vi "DrawBuoy.vi"(2 "Array":dbl[][](array[numeric]), 3 "2D Picture":picture) -> (0 "new picture":picture)   [LabVIEW 2012]
doc: "Draws a magenta circle at the curretn (x,y) coordinates of the Robot in the current mission definition file.\nInputs:\nPicture to draw on\nCluster X\n y coordinates of robot\nOutput:\nmodified picture"
panel:
  # "Draws a circle at the current x,y coordinates of the robot"
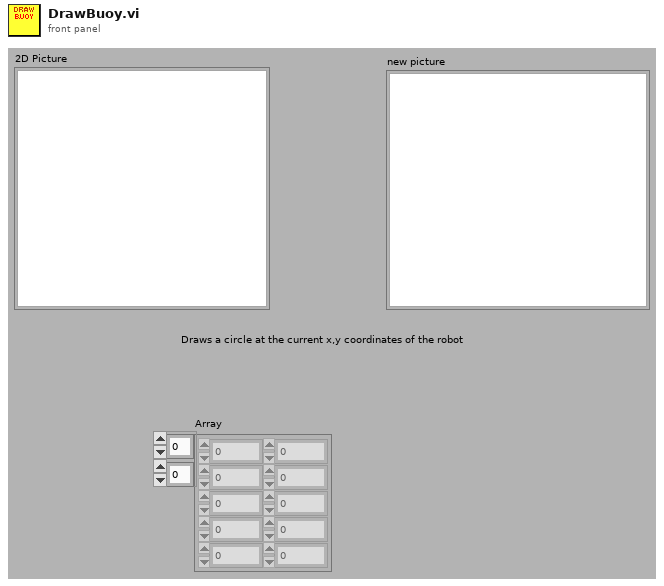
[diagram p1: front panel]
types:
  T1 = cluster{"Width":u16, "Style":enum32{"Solid", "Dash", "Dot", "DashDot", "DashDotDot"}}
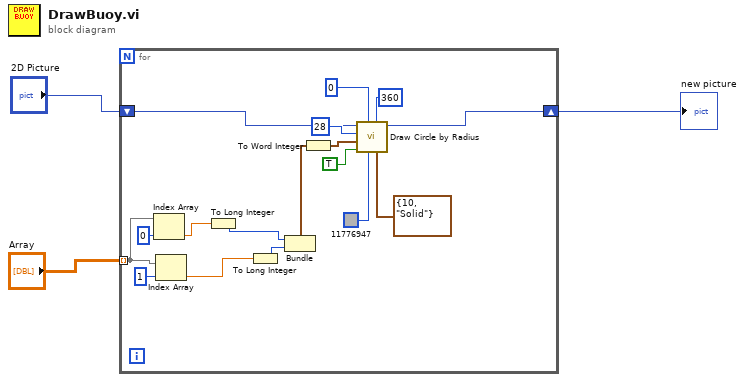
[diagram p0: block diagram]
diagram:
  n1 = for {
    shift-right: [w9] -> w2
    shift-left: "2D Picture" -> [w14]
    tunnel: "Array" -> [w6] mode=indexing
    n2 = Index Array(array=w6, index=0) -> (element=w5:dbl)
    n3 = Index Array(array=w6, index=1) -> (element=w4:dbl)
    n4 = To Long Integer(number=w5) -> (32bit integer=w12:i32)
    n5 = To Long Integer(number=w4) -> (32bit integer=w11:i32)
    n6 = Bundle(w12, w11) -> (w10:cluster{i32, i32})  [unwired: 1 in]
    n7 = To Word Integer(number=w10) -> (16bit integer=w20:cluster{i16, i16})
    n8 = call <vilib>:"Draw Circle by Radius.vi"("pen"=T1 {"Width"=10, "Style"=enum."Solid"}, "arc size(360)"=i16 360, "color(black)"=u32 11776947, "start angle(0)"=i16 0, "fill?(F)"=TRUE, "pixel center"=w20, "radius"=i16 28, "picture"=w14) -> ("new picture"=w9:picture)  [unwired: 3 in]
  }
  "new picture" <- w2
